vi "Toggle By Name.vi"(8 "error in":errorcluster, 9 "State":bool, 10 "Name":string, 11 "DAQ970 in":refnum<class "DAQ970.lvclass">) -> (0 "error out":errorcluster, 3 "DAQ970 out":refnum<class "DAQ970.lvclass">)   [LabVIEW 2019, in "DAQ970.lvlib" / "DAQ970.lvclass"]
uses:
  Library/DAQ970.lvclass
  C:/Users/Public/Documents/Development/builds/Instruments/Instruments.lvlibp/Library/Instruments.lvclass
  Library/DAQ970.lvclass/DAQ970.ctl
  builds/Instruments/Instruments.lvlibp/Private/Polymorphic/Special/Event from Boolean.vi
  builds/Instruments/Instruments.lvlibp/Accessors/Command with Logging.vi
  builds/Instruments/Instruments.lvlibp/Library/Instruments.lvclass
  builds/Instruments/Instruments.lvlibp
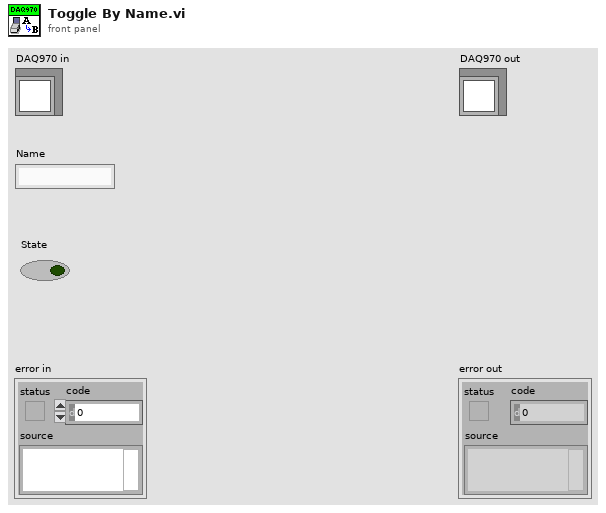
[diagram p1: front panel]
types:
  T1 = cluster{"Timestamp":timestamp, "Description":string, "Data":string}
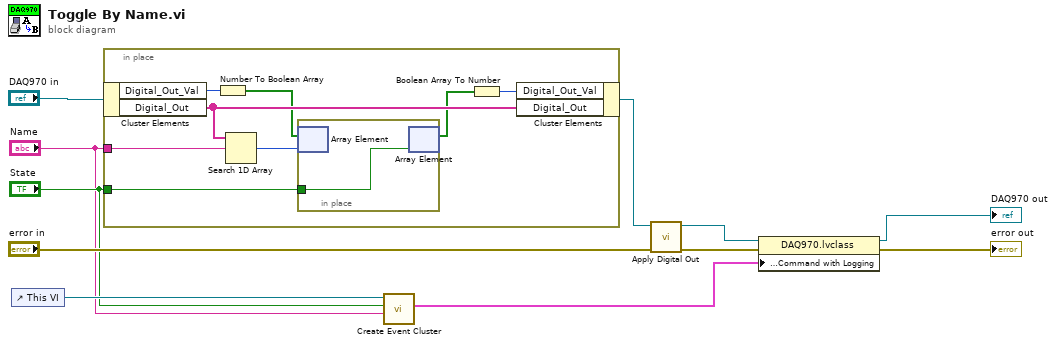
[diagram p0: block diagram]
diagram:
  n1 = control-ref of="This VI"() -> (w8:refnum<vi>)
  n2 = in-place {
    in-place-border: "Name" -> [w18]
    in-place-border: "State" -> [w12]
    n3 = in-place-cluster #1("DAQ970 in") -> ("Digital_Out_Val"=w17:u32, "Digital_Out"=w19:string[])
    n4 = Number To Boolean Array(number=w17) -> (Boolean array=w14:bool[])
    n5 = Search 1D Array(1D array=w19, element=w18) -> (index of element=w15:i32)  [unwired: 1 in]
    n6 = in-place {
      in-place-border: w12 -> [w20]
      n7 = in-place-array #2(w14, w15) -> ()  [unwired: 1 out]
      n8 = in-place-array #2(w20) -> (w13:bool[])  [unwired: 1 out]
    }
    n9 = Boolean Array To Number(Boolean array=w13) -> (number=w16:u32)
    n10 = in-place-cluster #1("Digital_Out_Val"=w16, "Digital_Out"=w19) -> (w10:refnum<class "DAQ970.lvclass">)
  }
  n11 = call-poly "Create Event Cluster.vi"("Name"="Name", "Value"="State", "VI Refnum"=w8) -> ("Event Data"=w1:T1)  [unwired: 8 in]
  n12 = call "Apply Digital Out.vi"("error in"="error in", "DAQ970 in"=w10) -> ("error out"=w4:errorcluster, "DAQ970 out"=w5:refnum<class "DAQ970.lvclass">)  [unwired: 8 in]
  n13 = property class="DAQ970.lvclass"(reference=w5, error in=w4, "Accessors:Logging:Command with Logging"=w1) -> (reference out=→"DAQ970 out":refnum<class "DAQ970.lvclass">, error out=→"error out":errorcluster)
